vi "Execute Kernel Advanced.vi"(6 "Local Work Size":T1 {"Width" min=1; "Height" min=1; "Depth" min=1}, 7 "Global Offset":T1 {"Width" min=1; "Height" min=1; "Depth" min=1}, 8 "Error In":errorcluster, 9 "Kernel Handle":T2, 10 "Thread Dimensions":T1={"Depth"=1, "Height"=1, "Width"=1} {"Width" min=1; "Height" min=1; "Depth" min=1}, 11 "Device In":T3) -> (0 "Error Out":errorcluster, 2 "Kernel Handle out":T2, 3 "Device Out":T3, 4 "Time in ms":dbl)   [LabVIEW 2012]
doc: "Executes a kernel after all the arguments have been set. The width, height, and depth of each respective dimension depends on the type of kernel being executed. It is recommended to read the OpenCL standard to best know how to use these. At a minimum, the user <b>must</b> set the <b>Thread Dimensions</b> parameters and leave the others to the default of {0,0,0}."
uses:
  Non-User VIs/Controls/Device ID.ctl
  Non-User VIs/Controls/Kernel Handle.ctl
  User Controls/Array Dimensions.ctl
  Non-User VIs/Error Checking/Add Error Functional Global.vi
  OpenCLV x64.lvlib
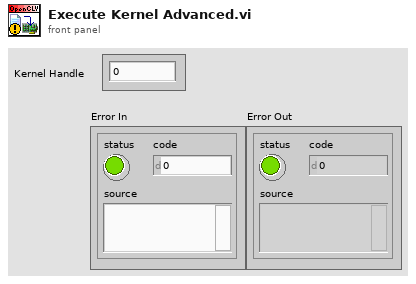
[diagram p1: front panel]
types:
  T1 = typedef "Array Dimensions.ctl" = cluster{"Depth":u64, "Height":u64, "Width":u64}
  T2 = typedef "OpenCLV x64.lvlib/Kernel Handle.ctl" = u64
  T3 = typedef "OpenCLV x64.lvlib/Device ID.ctl" = u64
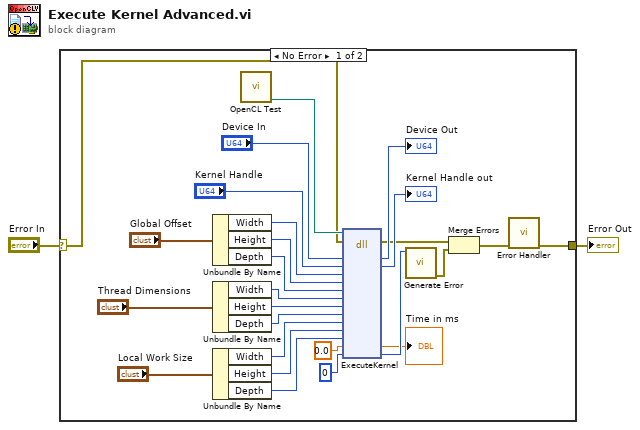
[diagram p0: block diagram]
diagram:
  n1 = case shown="No Error" "Error In" {
    selector: "Error In" -> [w3 w29]
    tunnel: [w7 w29] -> w1
    frame No Error {
      n2 = Unbundle By Name("Global Offset") -> ("Width"=w14:u64, "Height"=w15:u64, "Depth"=w16:u64)
      n3 = Unbundle By Name("Thread Dimensions") -> ("Width"=w24:u64, "Height"=w23:u64, "Depth"=w22:u64)
      n4 = Unbundle By Name("Local Work Size") -> ("Width"=w12:u64, "Height"=w11:u64, "Depth"=w10:u64)
      n5 = call "OpenCL Test.vi"() -> ("DLL To Use"=w8:path)  [unwired: 11 in]
      n6 = dll-call lib="C:/Users/bme-amcelroy-la/Desktop/OpenCLV/trunk/OpenCLV_x64_1.0/OpenCLV_x64.dll" fn="ExecuteKernel"(path in=w8, error in=w3, "Device In"="Device In", "Kernel"="Kernel Handle", "Global Width Offset"=w14, "Global Height Offset"=w15, "Global Depth Offset"=w16, "Global Width"=w24, "Global Height"=w23, "Global Depth"=w22, "Local Width"=w12, "Local Height"=w11, "Local Depth"=w10, "Time"=0.0, "Error"=0) -> (error out=w5:errorcluster, "Device In"=→"Device Out":u64, "Kernel"=→"Kernel Handle out":u64, "Time"=→"Time in ms":dbl, "Error"=w19:i32)  [unwired: 11 in, 1 out]
      n7 = call "Generate Error.vi"("Error"=w19) -> ("error out"=w6:errorcluster)  [unwired: 10 in]
      n8 = Merge Errors(w5, w6) -> (w4:errorcluster)
      n9 = call-poly "Error Handler.vi"("Error In"=w4) -> ("Error Out"=w7:errorcluster)  [unwired: 10 in]
    }
    frame Error {
    }
  }
  "Error Out" <- w1
